vi "XML Attribute String.vi"(9 "Value":string, 10 "Name":string, 11 "Prefix":string) -> (3 "Attribute string":string)   [LabVIEW 2012]
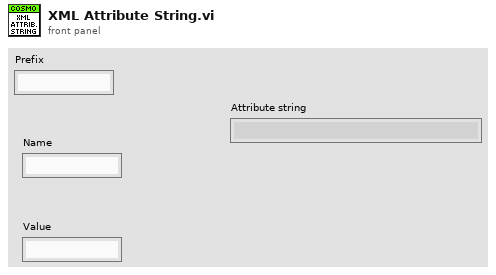
[diagram p1: front panel]
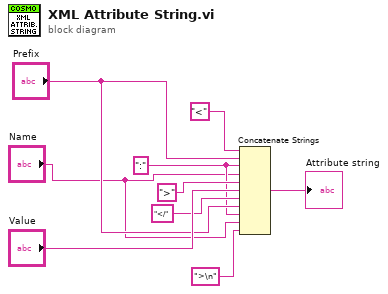
[diagram p0: block diagram]
diagram:
  w4 = ":" ("string")
  n1 = Concatenate Strings("<" ("string"), "Prefix", w4, "Name", ">" ("string"), "Value", "</" ("string"), "Prefix", w4, "Name", ">\n" ("string")) -> (→"Attribute string":string)
